vi "Actor Core.vi"(8 "error in":errorcluster, 11 "Controller in":refnum<class "Controller.lvclass">) -> (0 "error out":errorcluster, 3 "Controller out":refnum<class "Actor.lvclass">)   [LabVIEW 2023, in "MVC Actors.lvlib" / "Controller.lvclass"]
doc: "(<B>Filename</B>: Actor Framework.lvlib:Actor.lvclass:Actor Core.vi)\n\nReceives messages to the actor, reacts to them, and initiates any error handling that may shut the actor down.\n\nDescendant classes may override this VI to append parallel tasks for the actor to complete while it handles messages. Overrides use the Call Parent Method node."
uses:
  Controller.lvclass
  <vilib>/ActorFramework/Actor/Actor.lvclass
  <vilib>/LS Instruments AG/Async Methods Actor/Async Methods Actor/Async Methods Actor/Async Methods Actor.lvclass
  Controller.lvclass/Controller.ctl
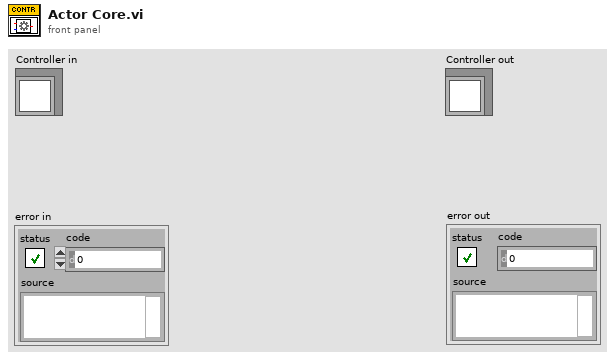
[diagram p1: front panel]
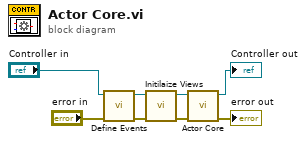
[diagram p0: block diagram]
diagram:
  n1 = call-dynamic "Define Events.vi"("error in (no error)"="error in", "Controller in"="Controller in") -> ("error out"=w2:errorcluster, "Controller out"=w1:refnum<class "Controller.lvclass">)  [unwired: 8 in]
  n2 = call-dynamic "Initilaize Views.vi"("error in (no error)"=w2, "Controller in"=w1) -> ("error out"=w3:errorcluster, "Controller out"=w5:refnum<class "Controller.lvclass">)  [unwired: 8 in]
  n3 = call-parent "Actor Core.vi"("error in"=w3, "Actor in"=w5) -> ("error out"=→"error out":errorcluster, "Actor out"=→"Controller out":refnum<class "Actor.lvclass">)  [unwired: 8 in]
